vi "Enable RTM Delete Logic.vi"(8 "error in (no error)":errorcluster, 9 "Sel.ItemNames":string[](array[string]), 10 "Running Tests":T1, 11 "Menu in":refnum<k9>) -> (0 "error out":errorcluster, 3 "Menu out":refnum<k9>)   [LabVIEW 2011]
uses:
  Controls/ListBox Test Record.ctl
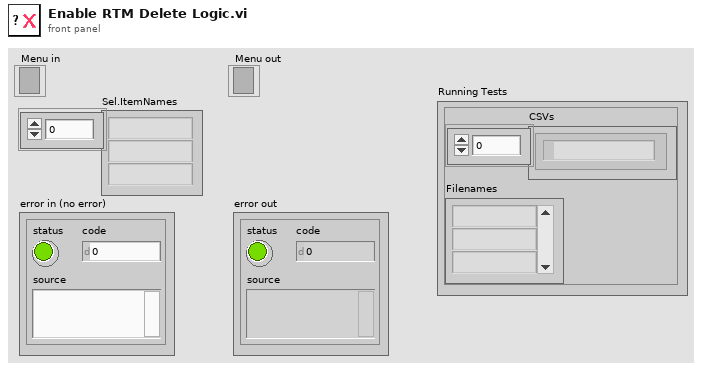
[diagram p1: front panel]
types:
  T1 = typedef "ListBox Test Record.ctl" = cluster{"CSVs":path[], "Filenames":string[]}
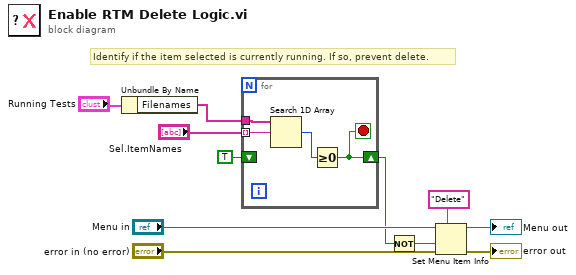
[diagram p0: block diagram]
diagram:
  # "Identify if the item selected is currently running. If so, prevent delete."
  n1 = Unbundle By Name("Running Tests") -> ("Filenames"=w4:string[])
  n2 = for {
    tunnel: "Sel.ItemNames" -> [w14] mode=indexing
    tunnel: w4 -> [w15]
    shift-right: [w12] -> w3
    shift-left: TRUE -> [_]
    stop <- w12 stop-if-true
    n3 = Search 1D Array(1D array=w15, element=w14) -> (index of element=w13:i32)  [unwired: 1 in]
    n4 = Greater Or Equal To 0?(x=w13) -> (x >= 0?=w12:bool)
  }
  n5 = Not(x=w3) -> (.not. x?=w2:bool)
  n6 = Set Menu Item Info(7:"Delete" ("item tag"), 8:"error in (no error)", 9:w2, 11:"Menu in") -> (0:→"error out":errorcluster, 3:→"Menu out":refnum<k9>)  [unwired: 3 in]
